vi "35Cl + 37Cl measure stable current.vi"(6 "measure transmission?":bool=TRUE, 7 "na/V 2":dbl=1000.0, 8 "error in":errorcluster, 9 "measure ss":bool, 10 "field change wait(s)":u32=5, 11 "na/V":dbl=500.0) -> (0 "error out":errorcluster, 1 "stable current 2":dbl format="%.2f", 3 "stable current":dbl format="%.2f", 4 "inj current":dbl format="%#_6e", 5 "INJ ss ratio":dbl format="%#_6e")   [LabVIEW 2016]
uses:
  stable controls/stable cluster.ctl
  kubley/data acquisition 2009/beamline/controls/stable state combo.ctl
panel:
  in  "Start.Delay":dbl=2.0 format="%#_13g"
  in  "Charge State":dbl=3.0
  out "stable 1":dbl[](graph)
  in  "stable data in":T1={"injector current"=1.0, "offset current"=1.0, "ss inj ratio"=1.0, "ss offset ratio"=1.0, "transmission"=1.0, "2nd offset current"=1.0}
  out "stable data out":T1={"injector current"=1.0, "offset current"=1.0, "ss inj ratio"=1.0, "ss offset ratio"=1.0, "transmission"=1.0, "2nd offset current"=1.0}
  out "stable 2":dbl[](graph)
  in  "inj current 4":dbl
  out "inj current 3":dbl format="%#_6e"
  in  "inj current 2":dbl
  out "step":string
  in  "measure stable":bool
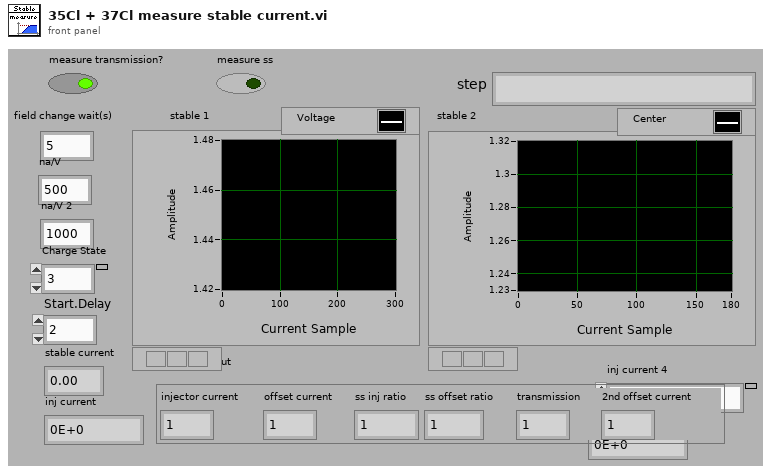
[diagram p1: front panel]
types:
  T1 = typedef "stable cluster.ctl" = cluster{"injector current":dbl, "offset current":dbl, "ss inj ratio":dbl, "ss offset ratio":dbl, "transmission":dbl, "2nd offset current":dbl}
  T2 = typedef "stable state combo.ctl" = string
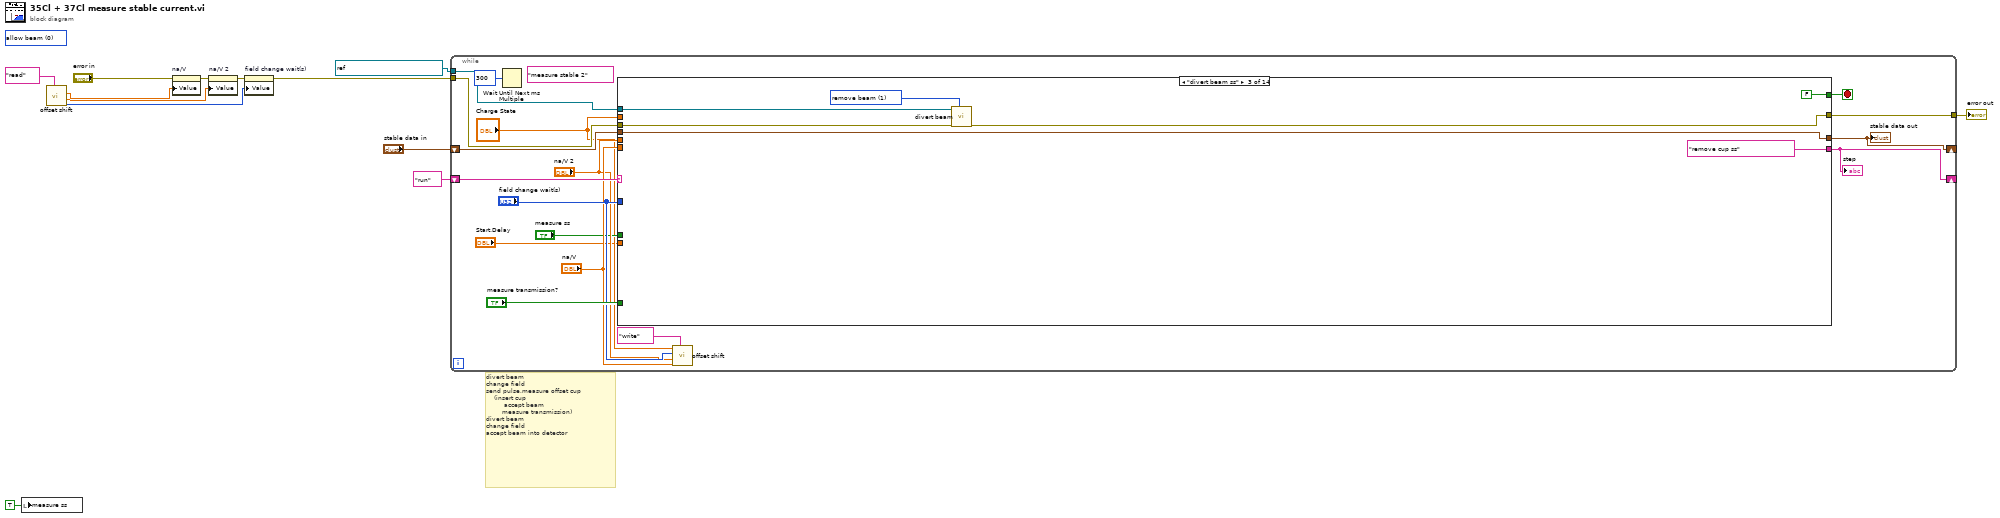
[diagram p0: block diagram]
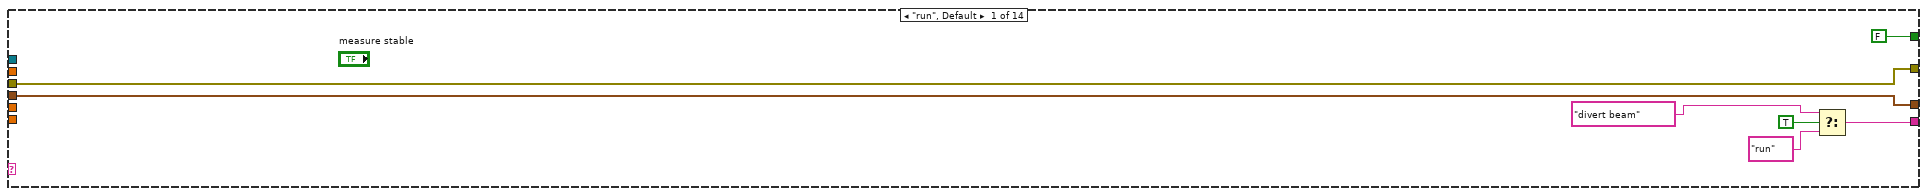
[diagram p2: hidden frame]
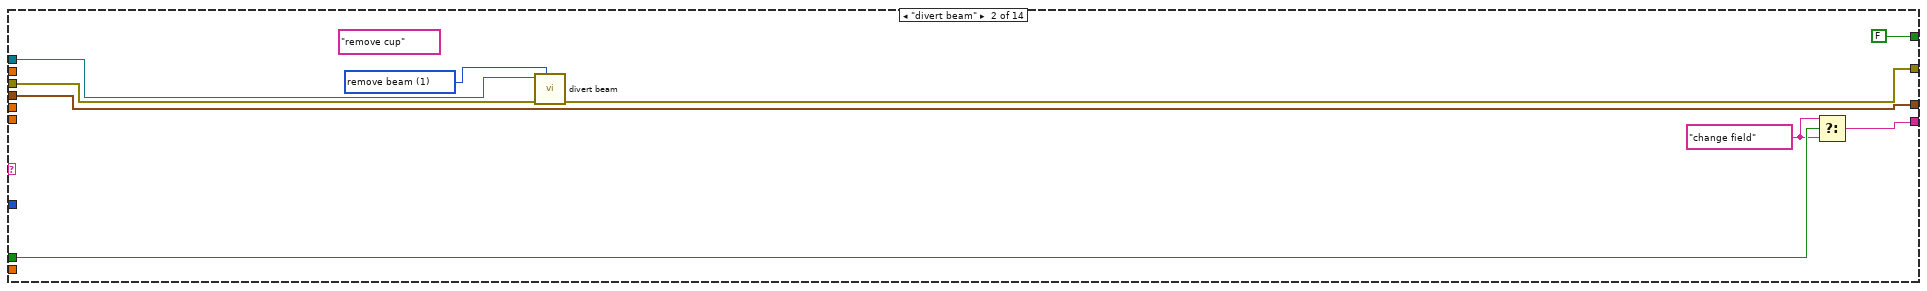
[diagram p3: hidden frame]
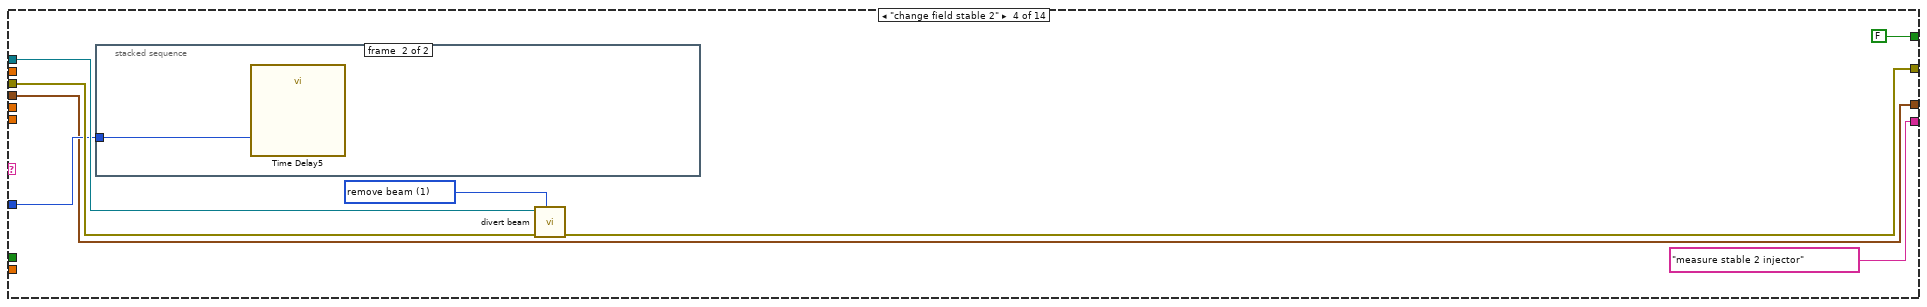
[diagram p4: hidden frame]
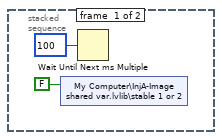
[diagram p5: hidden frame]
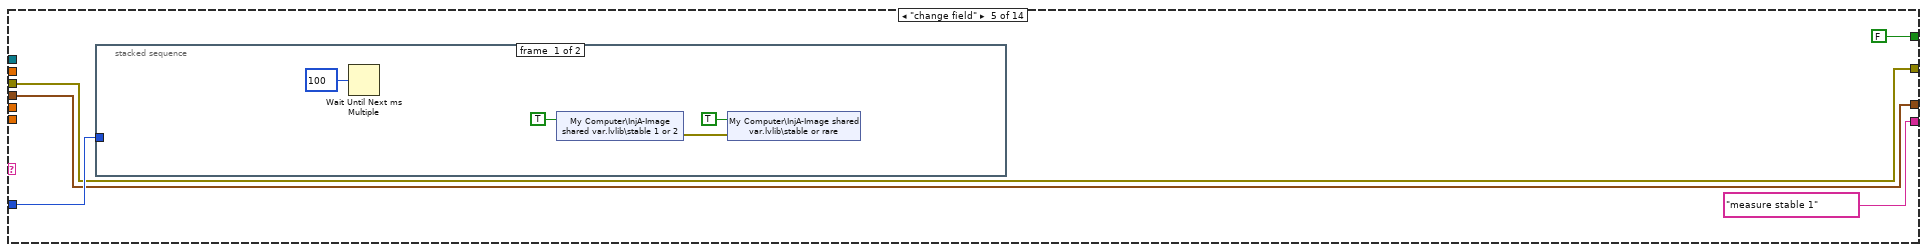
[diagram p6: hidden frame]
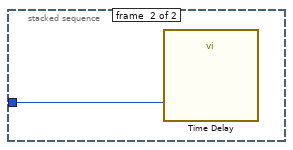
[diagram p7: hidden frame]
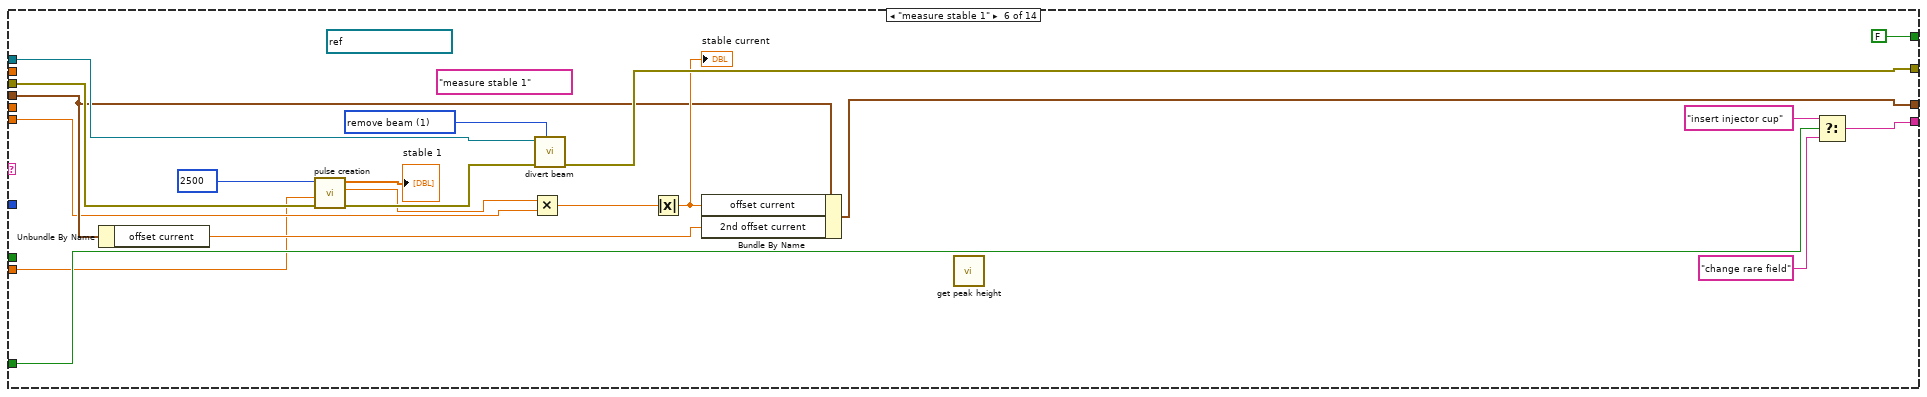
[diagram p8: hidden frame]
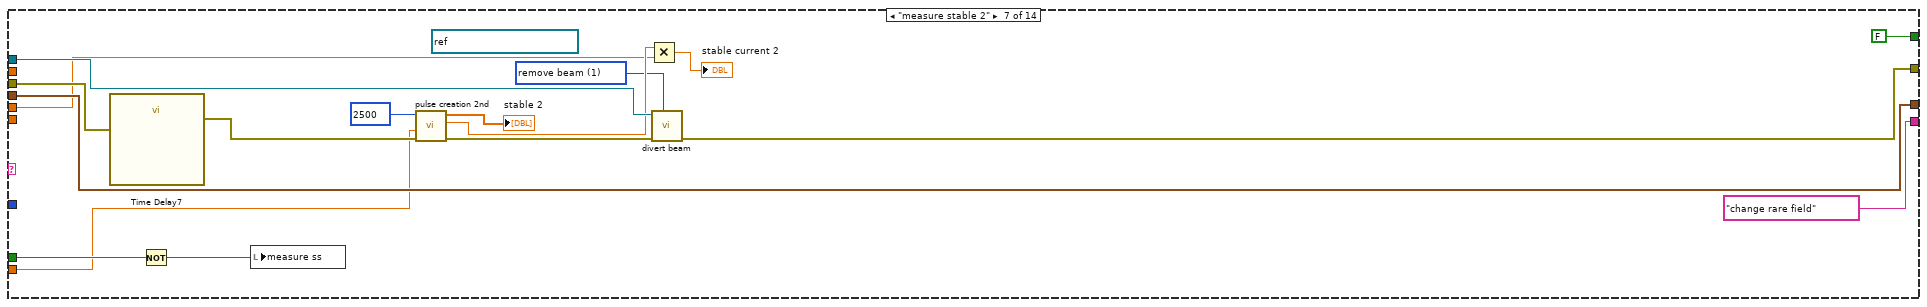
[diagram p9: hidden frame]
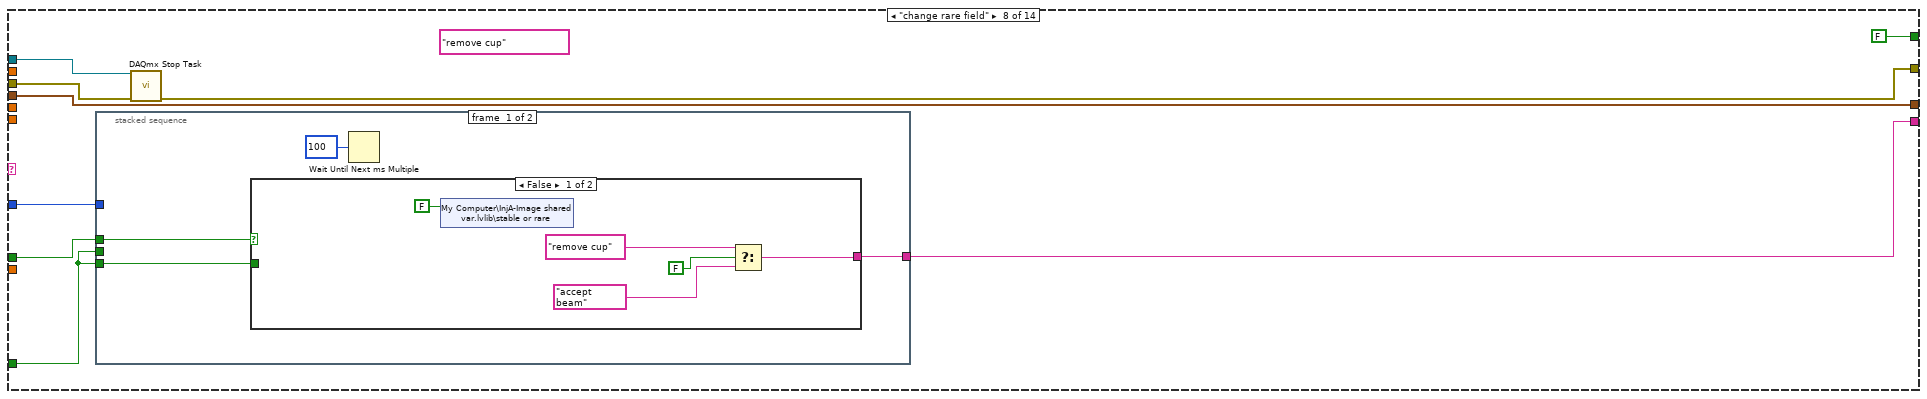
[diagram p10: hidden frame]
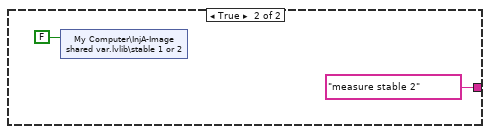
[diagram p11: hidden frame]
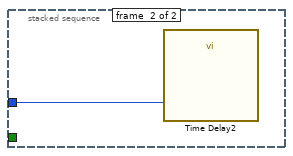
[diagram p12: hidden frame]
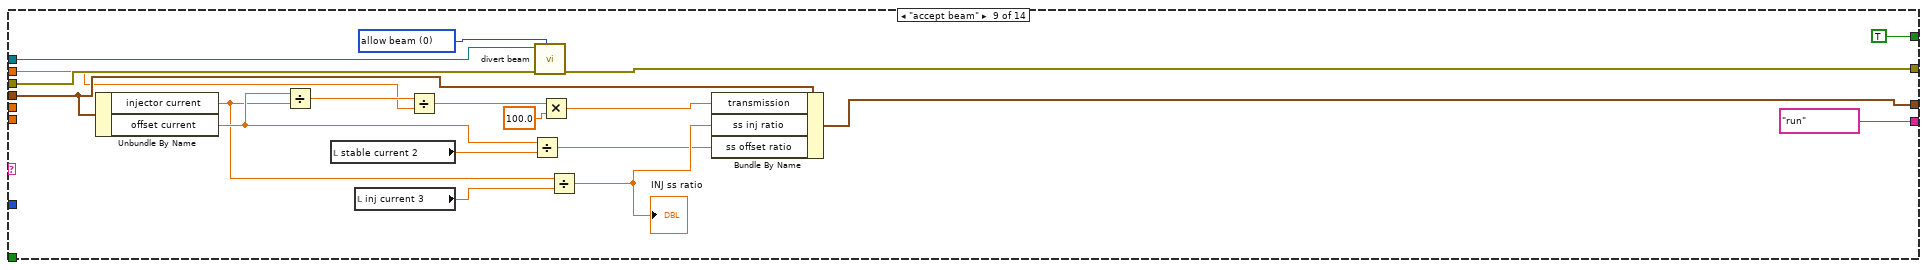
[diagram p13: hidden frame]
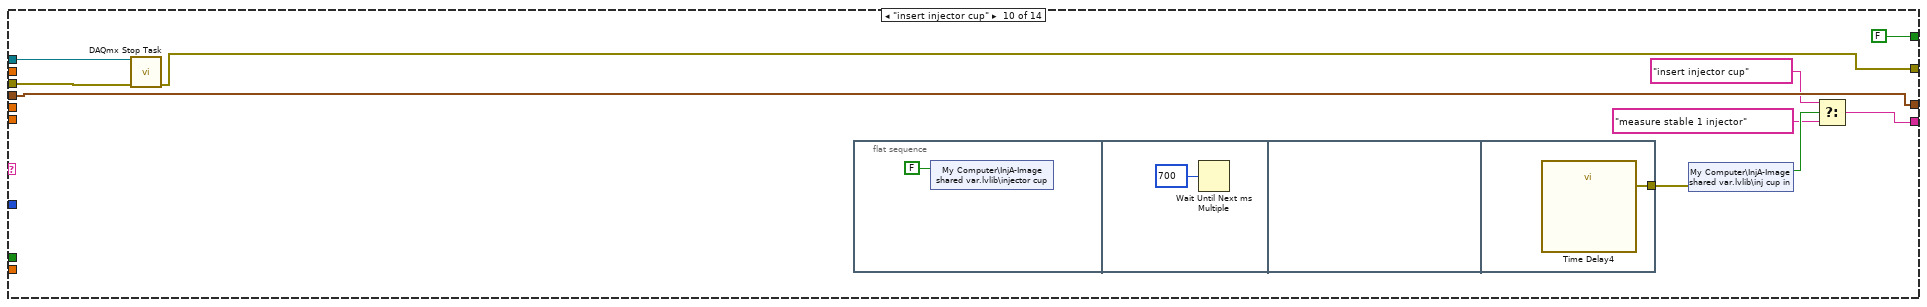
[diagram p14: hidden frame]
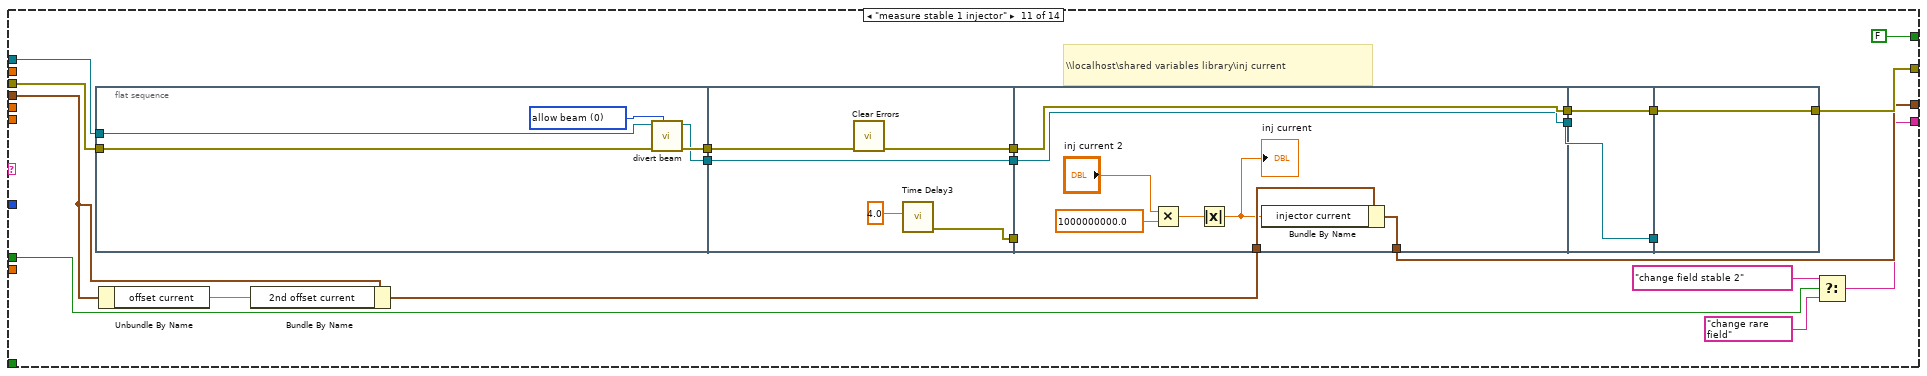
[diagram p15: hidden frame]
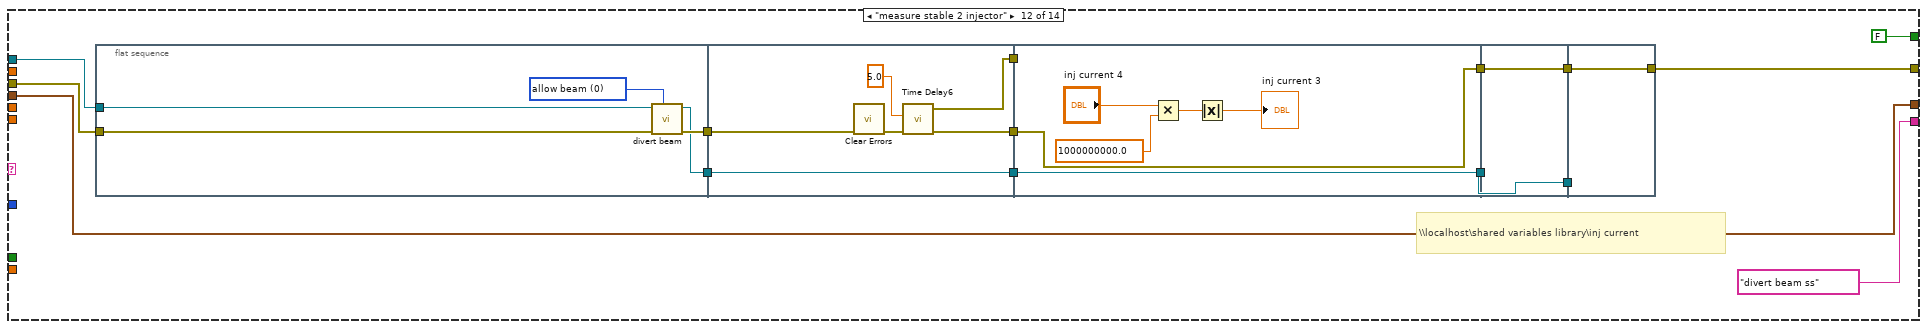
[diagram p16: hidden frame]
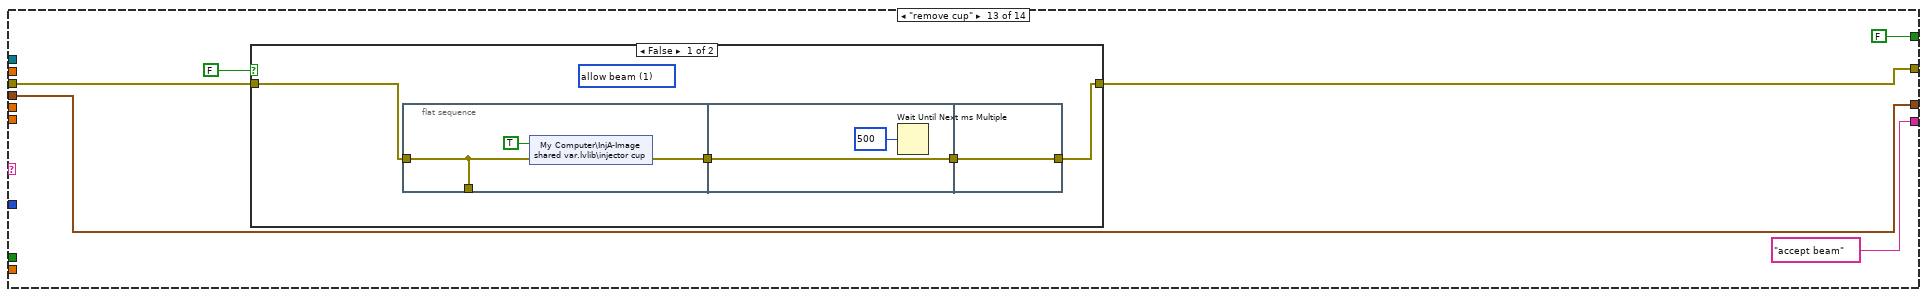
[diagram p17: hidden frame]
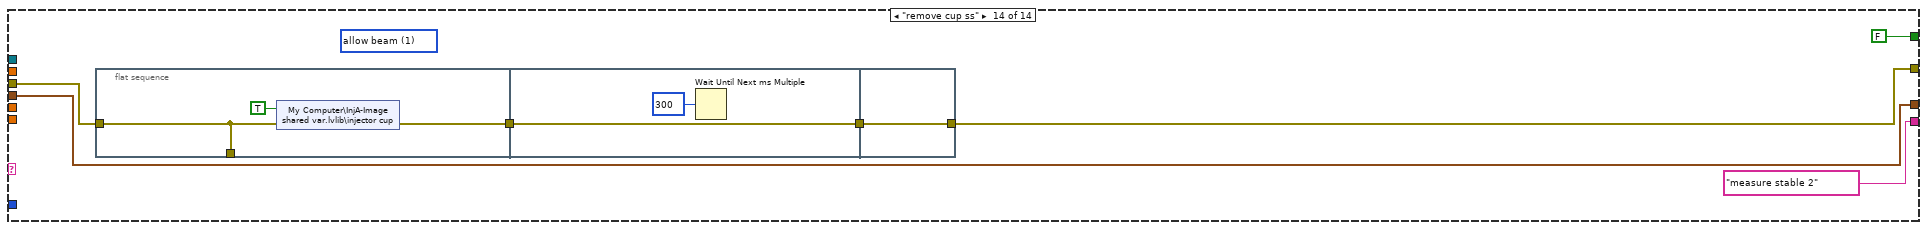
[diagram p19: hidden frame]
diagram:
  (unwired) u16 0 items=["allow beam", "remove beam"] ("divert beam? 2")
  # "divert beam\nchange field\nsend pulse,measure offset cup\n    (insert cup\n         accept beam\n        measure transmission)\ndivert beam\nchange field\naccept beam into detector"
  n1 = local write "measure ss"(TRUE ("measure ss")) -> ()
  n2 = call "offset shift.vi"("read writ"="read") -> ("field change wait(s) out"=w6:u32, "na/V 2out"=w7:dbl, "na/V out"=w8:dbl)  [unwired: 7 in, 1 out]
  n3 = property on="na/V" class="DigNum (strict)"(error in="error in", "Value"=w8) -> (error out=w5:errorcluster)  [unwired: 1 in, 1 out]
  n4 = property on="na/V 2" class="DigNum (strict)"(error in=w5, "Value"=w7) -> (error out=w4:errorcluster)  [unwired: 1 in, 1 out]
  n5 = property on="field change wait(s)" class="DigNum (strict)"(error in=w4, "Value"=w6) -> (error out=w3:errorcluster)  [unwired: 1 in, 1 out]
  n6 = while {
    shift-right: [w29] -> _
    shift-left: T2 "run" ("stable measurement type") -> [w30]
    tunnel: refnum<k21> "stable current output" ("task/channels in") -> [w28]
    tunnel: [w26] -> w11
    tunnel: w3 -> [w25]
    shift-right: [w21] -> _
    shift-left: "stable data in" -> [w22]
    stop <- w24 stop-if-true
    (unwired) T2 "measure stable 2" ("stable measurement type")
    n7 = Wait Until Next ms Multiple(millisecond multiple=u32 300) -> ()  [unwired: 1 out]
    n8 = case shown="\"divert beam ss\"" w30 {
      tunnel: [w35 w41 T2 "remove cup ss" ("stable measurement type") T2 "measure stable 2 injector" ("stable measurement type") T2 "measure stable 1" ("stable measurement type") w85 T2 "change rare field" ("stable measurement type") w113 T2 "run" ("stable measurement type") w155 w165 T2 "divert beam ss" ("stable measurement type") T2 "accept beam" ("stable measurement type") T2 "measure stable 2" ("stable measurement type")] -> w29
      tunnel: w28 -> [_ w46 w53 w61 _ w90 w108 w118 w151 w160 w182 w219 _ _]
      tunnel: "field change wait(s)" -> [_ _ _ w56 w68 _ _ w120 _ _ _ _ _ _]
      tunnel: [FALSE ("stop") FALSE ("stop") FALSE ("stop") FALSE ("stop") FALSE ("stop") FALSE ("stop") FALSE ("stop") FALSE ("stop") TRUE ("stop") FALSE ("stop") FALSE ("stop") FALSE ("stop") FALSE ("stop") FALSE ("stop")] -> w24
      tunnel: [w32 w44 w51 w58 w66 w87 w106 w116 w147 w158 w173 w210 w243 w261] -> w26
      tunnel: w25 -> [w32 w43 w50 w57 w66 w91 w102 w117 w148 w159 w179 w216 w244 w262]
      tunnel: "measure transmission?" -> [_ _ _ _ _ w89 _ w114 _ _ _ _ _ _]
      tunnel: "measure ss" -> [_ w42 _ _ _ _ w104 w115 _ _ w172 _ _ _]
      tunnel: w22 -> [w31 w38 w47 w54 w65 w79 w97 w112 w143 w154 w169 w208 w241 w258]
      tunnel: [w31 w38 w47 w54 w65 w80 w97 w112 w142 w154 w171 w208 w241 w258] -> w21
      tunnel: "Charge State" -> [_ _ _ _ _ _ _ _ w138 _ _ _ _ _]
      tunnel: "na/V" -> [_ _ _ _ _ w77 _ _ _ _ _ _ _ _]
      tunnel: "na/V 2" -> [_ _ _ _ _ _ w96 _ _ _ _ _ _ _]
      tunnel: "Start.Delay" -> [_ _ _ _ _ w75 w95 _ _ _ _ _ _ _]
      frame "run", Default {
        n9 = Select(t=T2 "divert beam" ("stable measurement type"), s=TRUE, f=T2 "run" ("stable measurement type")) -> (s? t:f=w35:T2)
      }
      frame "divert beam" {
        w39 = u16 1 items=["allow beam", "remove beam"] ("divert beam? 2")
        (unwired) T2 "remove cup" ("stable measurement type")
        w40 = T2 "change field" ("stable measurement type")
        n10 = call "divert beam.vi"("divert beam?"=w39, "error in"=w43, "task/channels in"=w46) -> ("error out"=w44:errorcluster)  [unwired: 7 in, 1 out]
        n11 = Select(t=w40, s=w42, f=w40) -> (s? t:f=w41:T2)
      }
      frame "divert beam ss" {
        w48 = u16 1 items=["allow beam", "remove beam"] ("divert beam? 2")
        n12 = call "divert beam.vi"("divert beam?"=w48, "error in"=w50, "task/channels in"=w53) -> ("error out"=w51:errorcluster)  [unwired: 7 in, 1 out]
      }
      frame "change field stable 2" {
        w55 = u16 1 items=["allow beam", "remove beam"] ("divert beam? 2")
        n13 = stacked-sequence {
          tunnel: w56 -> [_ w64]
          frame #0 {
            n14 = shared-variable "My Computer\\InjA-Image shared var.lvlib\\stable 1 or 2"(FALSE ("stable or rare")) -> ()  [unwired: 1 in, 1 out]
            n15 = Wait Until Next ms Multiple(millisecond multiple=u32 100) -> ()  [unwired: 1 out]
          }
          frame #1 {
            n16 = call "Time Delay5"("Delay Time (s)"=w64) -> ()  [unwired: 10 in, 1 out]
          }
        }
        n17 = call "divert beam.vi"("divert beam?"=w55, "error in"=w57, "task/channels in"=w61) -> ("error out"=w58:errorcluster)  [unwired: 7 in, 1 out]
      }
      frame "change field" {
        n18 = stacked-sequence {
          tunnel: w68 -> [_ w74]
          frame #0 {
            n19 = Wait Until Next ms Multiple(millisecond multiple=u32 100) -> ()  [unwired: 1 out]
            n20 = shared-variable "My Computer\\InjA-Image shared var.lvlib\\stable 1 or 2"(TRUE ("stable or rare")) -> (error out=w70:errorcluster)  [unwired: 1 in]
            n21 = shared-variable "My Computer\\InjA-Image shared var.lvlib\\stable or rare"(TRUE ("stable or rare"), error in=w70) -> ()  [unwired: 1 out]
          }
          frame #1 {
            n22 = call "Time Delay"("Delay Time (s)"=w74) -> ()  [unwired: 10 in, 1 out]
          }
        }
      }
      frame "measure stable 1" {
        w82 = u16 1 items=["allow beam", "remove beam"] ("divert beam? 2")
        (unwired) refnum<k21> "stable currents" ("task/channels in")
        (unwired) T2 "measure stable 1" ("stable measurement type")
        n23 = Unbundle By Name(w79) -> ("offset current"=w78:dbl)
        n24 = call "pulse creation.vi"("error in"=w91, "Start.Delay"=w75, "chopper width(usec)"=u32 2500) -> ("error out"=w93:errorcluster, "mean"=w83:dbl, "Waveform Graph 2"=→"stable 1":dbl[])  [unwired: 4 in, 2 out]
        n25 = Multiply(x=w83, y=w77) -> (x*y=w84:dbl)
        n26 = call "divert beam.vi"("divert beam?"=w82, "error in"=w93, "task/channels in"=w90) -> ("error out"=w87:errorcluster)  [unwired: 7 in, 1 out]
        n27 = Absolute Value(x=w84) -> (abs(x)=w81:dbl)
        "stable current" <- w81
        n28 = Bundle By Name(cluster=w79, "offset current"=w81, "2nd offset current"=w78) -> (w80:T1)
        n29 = call "get peak height.vi"() -> ()  [unwired: 8 in, 4 out]
        n30 = Select(t=T2 "insert injector cup" ("stable measurement type"), s=w89, f=T2 "change rare field" ("stable measurement type")) -> (s? t:f=w85:T2)
      }
      frame "measure stable 2" {
        w98 = u16 1 items=["allow beam", "remove beam"] ("divert beam? 2")
        (unwired) refnum<k21> "secondary current" ("task/channels in")
        n31 = call "Time Delay7"("error in (no error)"=w102) -> ("error out"=w101:errorcluster)  [unwired: 10 in]
        n32 = Not(x=w104) -> (.not. x?=w103:bool)
        n33 = local write "measure ss"(w103) -> ()
        n34 = call "pulse creation 2nd.vi"("error in"=w101, "Start.Delay"=w95, "chopper width(usec)"=u32 2500) -> ("error out"=w110:errorcluster, "mean"=w99:dbl, "Waveform Graph"=→"stable 2":dbl[])  [unwired: 6 in]
        n35 = Multiply(x=w99, y=w96) -> (x*y=→"stable current 2":dbl)
        n36 = call "divert beam.vi"("divert beam?"=w98, "error in"=w110, "task/channels in"=w108) -> ("error out"=w106:errorcluster)  [unwired: 7 in, 1 out]
      }
      frame "change rare field" {
        (unwired) T2 "remove cup" ("stable measurement type")
        n37 = stacked-sequence {
          tunnel: w120 -> [_ w132]
          tunnel: w115 -> [w123 _]
          tunnel: w114 -> [w122 _]
          tunnel: w114 -> [_ _]
          tunnel: [w121 _] -> w113
          frame #0 {
            n38 = case shown="False" w123 {
              tunnel: w122 -> [_ _]
              tunnel: [w126 T2 "measure stable 2" ("stable measurement type")] -> w121
              frame False {
                n39 = shared-variable "My Computer\\InjA-Image shared var.lvlib\\stable or rare"(FALSE ("stable or rare")) -> ()  [unwired: 1 in, 1 out]
                n40 = Select(t=T2 "remove cup" ("stable measurement type"), s=FALSE ("stable or rare"), f=T2 "accept beam" ("stable measurement type")) -> (s? t:f=w126:T2)
              }
              frame True {
                n41 = shared-variable "My Computer\\InjA-Image shared var.lvlib\\stable 1 or 2"(FALSE ("stable or rare")) -> ()  [unwired: 1 in, 1 out]
              }
            }
            n42 = Wait Until Next ms Multiple(millisecond multiple=u32 100) -> ()  [unwired: 1 out]
          }
          frame #1 {
            n43 = call "Time Delay2"("Delay Time (s)"=w132) -> ()  [unwired: 10 in, 1 out]
          }
        }
        n44 = call <vilib>:"DAQmx Stop Task.vi"("task/channels in"=w118, "error in"=w117) -> ("error out"=w116:errorcluster)  [unwired: 12 in, 1 out]
      }
      frame "accept beam" {
        w145 = u16 0 items=["allow beam", "remove beam"] ("divert beam? 2")
        n45 = Unbundle By Name(w143) -> ("injector current"=w134:dbl, "offset current"=w135:dbl)
        n46 = Divide(x=w135, y=w134) -> (x/y=w144:dbl)
        n47 = local read "stable current 2"() -> (w136:dbl)
        n48 = local read "inj current 3"() -> (w146:dbl)
        n49 = Divide(x=w144, y=w138) -> (x/y=w141:dbl)
        n50 = Divide(x=w135, y=w136) -> (x/y=w133:dbl)
        n51 = call "divert beam.vi"("divert beam?"=w145, "error in"=w148, "task/channels in"=w151) -> ("error out"=w147:errorcluster)  [unwired: 7 in, 1 out]
        n52 = Multiply(x=w141, y=100.0) -> (x*y=w139:dbl)
        n53 = Divide(x=w134, y=w146) -> (x/y=w137:dbl)
        "INJ ss ratio" <- w137
        n54 = Bundle By Name(cluster=w143, "transmission"=w139, "ss inj ratio"=w137, "ss offset ratio"=w133) -> (w142:T1)
      }
      frame "insert injector cup" {
        n55 = call <vilib>:"DAQmx Stop Task.vi"("task/channels in"=w160, "error in"=w159) -> ("error out"=w158:errorcluster)  [unwired: 12 in, 1 out]
        n56 = flat-sequence {
          tunnel: [w164] -> w157
          frame #0 {
            n57 = shared-variable "My Computer\\InjA-Image shared var.lvlib\\injector cup"(FALSE ("injector cup")) -> ()  [unwired: 1 in, 1 out]
          }
          frame #1 {
            n58 = Wait Until Next ms Multiple(millisecond multiple=u32 700) -> ()  [unwired: 1 out]
          }
          frame #2 {
          }
          frame #3 {
            n59 = call "Time Delay4"() -> ("error out"=w164:errorcluster)  [unwired: 11 in]
          }
        }
        n60 = shared-variable "My Computer\\InjA-Image shared var.lvlib\\inj cup in"(error in=w157) -> (w156:bool)  [unwired: 1 out]
        n61 = Select(t=T2 "insert injector cup" ("f"), s=w156, f=T2 "measure stable 1 injector" ("stable measurement type")) -> (s? t:f=w155:T2)
      }
      frame "measure stable 1 injector" {
        # "\\\\localhost\\shared variables library\\inj current"
        n62 = flat-sequence {
          tunnel: w182 -> [w190]
          tunnel: [w189] -> w183
          tunnel: [w187] -> w180
          tunnel: w179 -> [w188]
          tunnel: [w193] -> w184
          tunnel: w183 -> [w194]
          tunnel: [w195] -> w181
          tunnel: w180 -> [w195]
          tunnel: [w191] -> w174
          tunnel: [w203] -> w178
          tunnel: w184 -> [w203]
          tunnel: [w202] -> w176
          tunnel: w181 -> [w202]
          tunnel: w174 -> [_]
          tunnel: w168 -> [w201]
          tunnel: [w200] -> w171
          tunnel: w178 -> [w205]
          tunnel: [w205] -> w177
          tunnel: w176 -> [w204]
          tunnel: [w204] -> w175
          tunnel: w177 -> [w206]
          tunnel: w175 -> [_]
          tunnel: [w206] -> w173
          frame #0 {
            w186 = u16 0 items=["allow beam", "remove beam"] ("divert beam? 2")
            n63 = call "divert beam.vi"("divert beam?"=w186, "error in"=w188, "task/channels in"=w190) -> ("error out"=w189:errorcluster, "task out"=w187:refnum<k21>)  [unwired: 7 in]
          }
          frame #1 {
            n64 = call <vilib>:"Clear Errors.vi"("error in (no error)"=w194) -> ("error out"=w193:errorcluster)  [unwired: 5 in, 1 out]
            n65 = call "Time Delay3"("Delay Time (s)"=4.0) -> ("error out"=w191:errorcluster)  [unwired: 10 in]
          }
          frame #2 {
            n66 = Multiply(x="inj current 2", y=1000000000.0) -> (x*y=w197:dbl)
            n67 = Absolute Value(x=w197) -> (abs(x)=w196:dbl)
            "inj current" <- w196
            n68 = Bundle By Name(cluster=w201, "injector current"=w196) -> (w200:T1)
          }
          frame #3 {
          }
          frame #4 {
          }
        }
        n69 = Unbundle By Name(w169) -> ("offset current"=w170:dbl)
        n70 = Bundle By Name(cluster=w169, "2nd offset current"=w170) -> (w168:T1)
        n71 = Select(t=T2 "change field stable 2" ("stable measurement type"), s=w172, f=T2 "change rare field" ("stable measurement type")) -> (s? t:f=w165:T2)
      }
      frame "measure stable 2 injector" {
        # "\\\\localhost\\shared variables library\\inj current"
        n72 = flat-sequence {
          tunnel: w219 -> [w226]
          tunnel: [w225] -> w220
          tunnel: [w223] -> w217
          tunnel: w216 -> [w224]
          tunnel: w220 -> [w230]
          tunnel: [w231] -> w218
          tunnel: w217 -> [w231]
          tunnel: [w227] -> w211
          tunnel: [w227] -> w207
          tunnel: [w237] -> w215
          tunnel: [w236] -> w213
          tunnel: w218 -> [w236]
          tunnel: w211 -> [_]
          tunnel: w207 -> [w237]
          tunnel: w215 -> [w239]
          tunnel: [w239] -> w214
          tunnel: w213 -> [w238]
          tunnel: [w238] -> w212
          tunnel: w214 -> [w240]
          tunnel: w212 -> [_]
          tunnel: [w240] -> w210
          frame #0 {
            w222 = u16 0 items=["allow beam", "remove beam"] ("divert beam? 2")
            n73 = call "divert beam.vi"("divert beam?"=w222, "error in"=w224, "task/channels in"=w226) -> ("error out"=w225:errorcluster, "task out"=w223:refnum<k21>)  [unwired: 7 in]
          }
          frame #1 {
            n74 = call <vilib>:"Clear Errors.vi"("error in (no error)"=w230) -> ("error out"=w228:errorcluster)  [unwired: 5 in, 1 out]
            n75 = call "Time Delay6"("error in (no error)"=w228, "Delay Time (s)"=5.0) -> ("error out"=w227:errorcluster)  [unwired: 9 in]
          }
          frame #2 {
            n76 = Multiply(x="inj current 4", y=1000000000.0) -> (x*y=w234:dbl)
            n77 = Absolute Value(x=w234) -> (abs(x)=→"inj current 3":dbl)
          }
          frame #3 {
          }
          frame #4 {
          }
        }
      }
      frame "remove cup" {
        n78 = case shown="False" FALSE {
          tunnel: w244 -> [w248 w257]
          tunnel: [w247 w257] -> w243
          frame False {
            (unwired) u16 1 items=["divert beam", "allow beam"] ("divert beam? 2")
            n79 = flat-sequence {
              tunnel: [w251] -> _
              tunnel: w248 -> [w251]
              tunnel: [w252] -> w250
              tunnel: [w254] -> w249
              tunnel: w250 -> [w254]
              tunnel: w249 -> [w256]
              tunnel: [w256] -> w247
              frame #0 {
                n80 = shared-variable "My Computer\\InjA-Image shared var.lvlib\\injector cup"(TRUE ("injector cup"), error in=w251) -> (error out=w252:errorcluster)
              }
              frame #1 {
                n81 = Wait Until Next ms Multiple(millisecond multiple=u32 500) -> ()  [unwired: 1 out]
              }
              frame #2 {
              }
            }
          }
          frame True {
          }
        }
      }
      frame "remove cup ss" {
        (unwired) u16 1 items=["divert beam", "allow beam"] ("divert beam? 2")
        n82 = flat-sequence {
          tunnel: [w265] -> _
          tunnel: w262 -> [w265]
          tunnel: [w266] -> w260
          tunnel: [w268] -> w259
          tunnel: w260 -> [w268]
          tunnel: w259 -> [w270]
          tunnel: [w270] -> w261
          frame #0 {
            n83 = shared-variable "My Computer\\InjA-Image shared var.lvlib\\injector cup"(TRUE ("injector cup"), error in=w265) -> (error out=w266:errorcluster)
          }
          frame #1 {
            n84 = Wait Until Next ms Multiple(millisecond multiple=u32 300) -> ()  [unwired: 1 out]
          }
          frame #2 {
          }
        }
      }
    }
    "step" <- w29
    "stable data out" <- w21
    n85 = call "offset shift.vi"("read writ"="write", "na/V"="na/V", "na/V 2"="na/V 2", "field change wait(s)"="field change wait(s)", "charge state"="Charge State") -> ()  [unwired: 3 in, 4 out]
  }
  "error out" <- w11
